vi "STATION_1_STATUS.vi"(8 "error in (no error)":errorcluster, 9 "FAULT NUMBER":i32, 10 "STATUS":string, 11 "Ctl Refnum":refnum<vi>) -> (0 "error out":errorcluster)   [LabVIEW 2017]
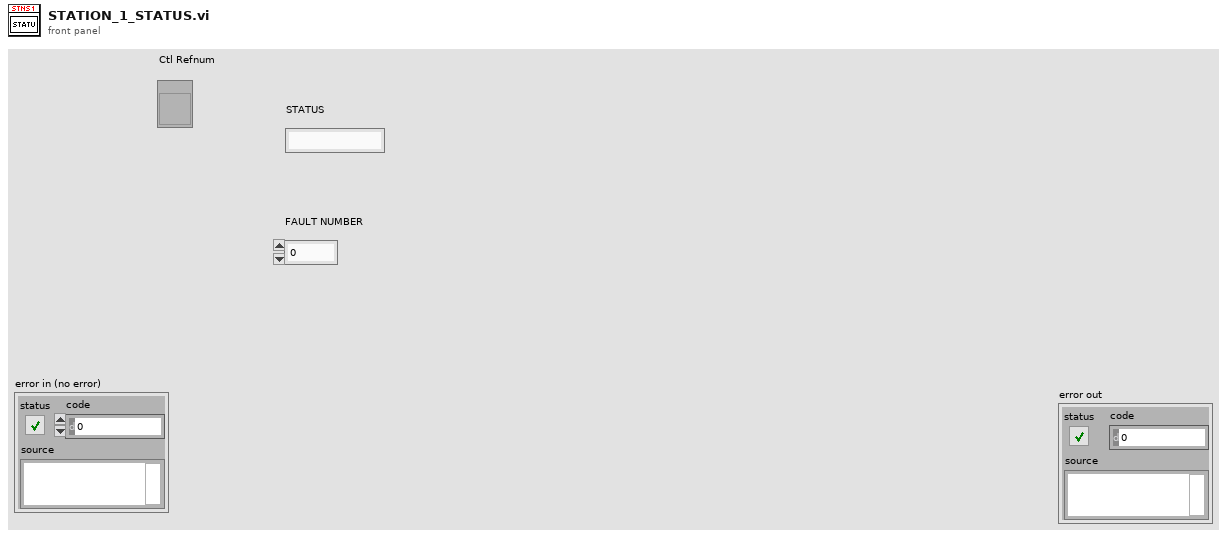
[diagram p1: front panel]
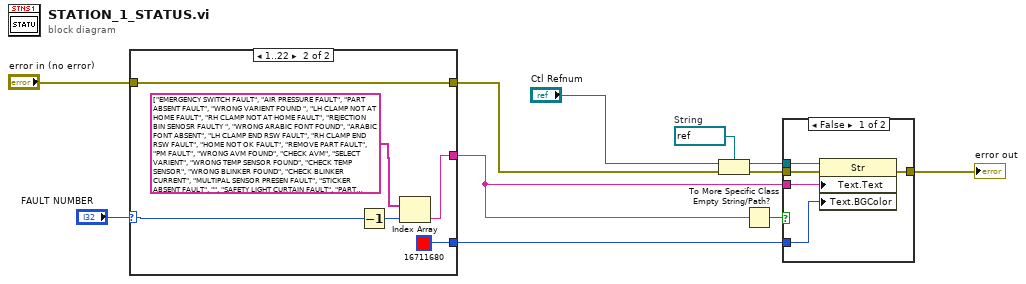
[diagram p0: block diagram]
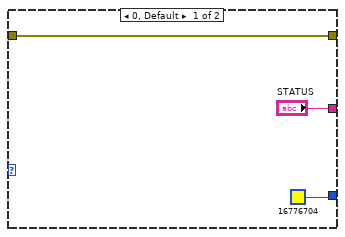
[diagram p3: hidden frame]
diagram:
  w11 = refnum<vi> refnum  # String
  n1 = case shown="1..22" "FAULT NUMBER" {
    selector: "FAULT NUMBER" -> [_ w19]
    tunnel: ["STATUS" w18] -> w3
    tunnel: [u32 16776704 ("Color Box 2") u32 16711680 ("Color Box 2")] -> w5
    tunnel: [w12 w16] -> w2
    tunnel: "error in (no error)" -> [w12 w16]
    frame 0, Default {
    }
    frame 1..22 {
      n2 = Decrement(x=w19) -> (x-1=w20:i32)
      n3 = Index Array(array=string[] ["EMERGENCY SWITCH FAULT", "AIR PRESSURE FAULT", "PART ABSENT FAULT", "WRONG VARIENT FOUND ", "LH CLAMP NOT AT HOME FAULT", "RH CLAMP NOT AT HOME FAULT", "REJECTION BIN SENOSR FAULTY ", "WRONG ARABIC FONT FOUND", "ARABIC FONT ABSENT", "LH CLAMP END RSW FAULT", "RH CLAMP END RSW FAULT", "HOME NOT OK FAULT", "REMOVE PART FAULT", "PM FAULT", "WRONG AVM FOUND", "CHECK AVM", "SELECT VARIENT", "WRONG TEMP SENSOR FOUND", "CHECK TEMP SENSOR", "WRONG BLINKER FOUND", "CHECK BLINKER CURRENT", "MULTIPAL SENSOR PRESEN FAULT", "STICKER ABSENT FAULT", "", "SAFETY LIGHT CURTAIN FAULT", "PART REJECT FOR POWER FAILURE\nWRONG TOOL LIFE", "WRONG TOOL LIFE", "WRONG PART SCAN", "SCAN NOT DONE"], index=w20) -> (element=w18:string)
    }
  }
  n4 = To More Specific Class(target class=w11, reference="Ctl Refnum", error in=w2) -> (specific class reference=w9:refnum<vi>, error out=w8:errorcluster)
  n5 = Empty String/Path?(string/path=w3) -> (empty?=w4:bool)
  n6 = case shown="False" w4 {
    tunnel: w9 -> [w25 _]
    tunnel: w8 -> [w24 w26]
    tunnel: [w23 w26] -> w7
    tunnel: w3 -> [w22 _]
    tunnel: w5 -> [w21 _]
    frame False {
      n7 = property class="Str"(reference=w25, error in=w24, "Text.Text"=w22, "Text.BGColor"=w21) -> (error out=w23:errorcluster)  [unwired: 1 out]
    }
    frame True {
    }
  }
  "error out" <- w7
